vi "Handle Error.vi"(8 "error in (no error)":errorcluster, 11 "PID Loop in":refnum<class "PID Loop.lvclass">) -> (0 "error out":errorcluster, 3 "PID Loop out":refnum<class "PID Loop.lvclass">, 4 "Exit?":bool)   [LabVIEW 2024, in "PID Loop.lvlib" / "PID Loop.lvclass"]
uses:
  PID Loop.lvclass
  PID Loop.lvclass/PID Loop.ctl
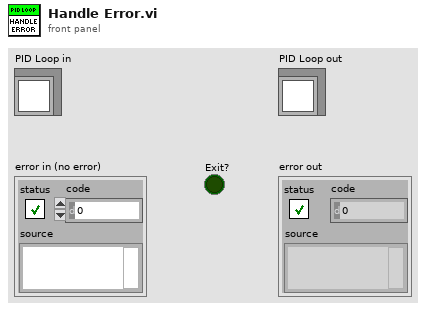
[diagram p1: front panel]
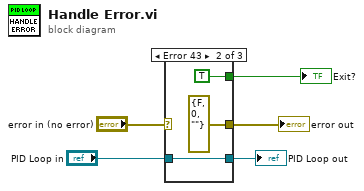
[diagram p0: block diagram]
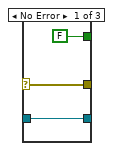
[diagram p2: hidden frame]
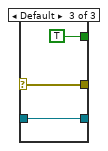
[diagram p3: hidden frame]
diagram:
  n1 = case shown="Error 43" "error in (no error)" {
    selector: "error in (no error)" -> [w7 _ w14]
    tunnel: [w7 errorcluster {"status"=FALSE, "code"=0, "source"=""} ("error IO") w14] -> w4
    tunnel: [w8 w9 w13] -> w2
    tunnel: "PID Loop in" -> [w8 w9 w13]
    tunnel: [FALSE TRUE TRUE] -> w1
    frame No Error {
    }
    frame Error {
    }
    frame Default {
    }
  }
  "error out" <- w4
  "PID Loop out" <- w2
  "Exit?" <- w1
